vi "BRig_FPGA_lick__v2.vi"(7 "Rising(F)_or_Falling(T)":bool, 8 "I_stateDetector_new":bool, 10 "counter":u32, 11 "I_stateDetector_prev":bool) -> (0 "output_I_lick":bool, 2 "output_counter":u32, 3 "output_I_stateDetector_prev":bool)   [LabVIEW 2014]
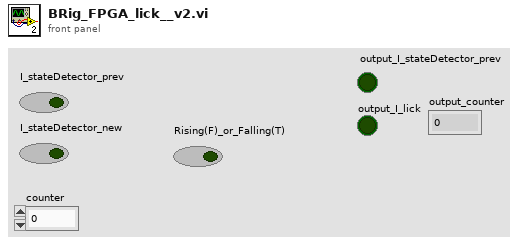
[diagram p1: front panel]
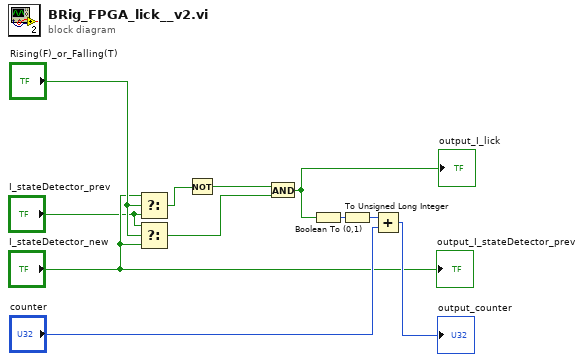
[diagram p0: block diagram]
diagram:
  n1 = Select(t="I_stateDetector_new", s="Rising(F)_or_Falling(T)", f="I_stateDetector_prev") -> (s? t:f=w2:bool)
  n2 = Select(t="I_stateDetector_prev", s="Rising(F)_or_Falling(T)", f="I_stateDetector_new") -> (s? t:f=w1:bool)
  n3 = Not(x=w2) -> (.not. x?=w5:bool)
  n4 = And(x=w5, y=w1) -> (x .and. y?=w10:bool)
  "output_I_lick" <- w10
  n5 = Boolean To (0,1)(Boolean=w10) -> (0, 1=w11:i16)
  n6 = To Unsigned Long Integer(number=w11) -> (unsigned 32bit integer=w9:u32)
  n7 = Add(x=w9, y="counter") -> (x+y=→"output_counter":u32)
  "output_I_stateDetector_prev" <- "I_stateDetector_new"
